vi "rotate_absolute.vi"(3 "error in (no error)":errorcluster, 4 "angle":i32, 5 "revolution":i32) -> (0 "error out":errorcluster)   [LabVIEW 2016]
uses:
  sa commands.ctl
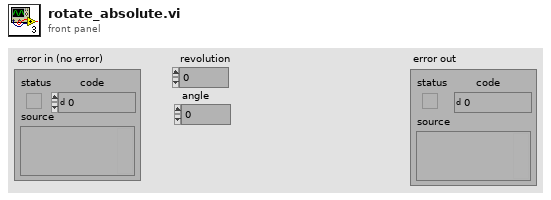
[diagram p1: front panel]
types:
  T1 = typedef "sa commands.ctl" = enum16{"read all", "set system index", "set x channel", "set y channel", "set rotation channel"}
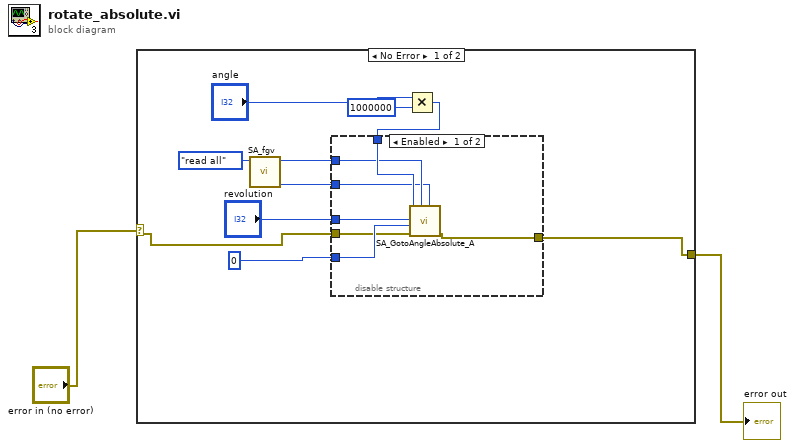
[diagram p0: block diagram]
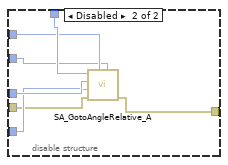
[diagram p2: hidden frame]
diagram:
  n1 = case shown="No Error" "error in (no error)" {
    selector: "error in (no error)" -> [w7 w27]
    tunnel: [w6 w27] -> w1
    frame No Error {
      n2 = call "SA_fgv.vi"("command"=sa_commands."read all") -> ("rotation channel"=w9:u32, "system index"=w10:u32)  [unwired: 3 in, 2 out]
      n3 = Multiply(x="angle", y=1000000) -> (x*y=w4:i32)
      n4 = disable-structure shown="Enabled" {
        disable-tunnel: u32 0 ("holdTime") -> [w19 w22]
        disable-tunnel: "revolution" -> [w18 w23]
        disable-tunnel: w4 -> [w17 w26]
        disable-tunnel: w10 -> [w16 w25]
        disable-tunnel: w9 -> [w15 w24]
        disable-tunnel: w7 -> [w14 w21]
        disable-tunnel: [w13 w20] -> w6
        frame Enabled {
          n5 = call <vilib>:"SA_GotoAngleAbsolute_A.vi"("channelIndex"=w15, "systemIndex"=w16, "error in (no error)"=w14, "holdTime"=w19, "revolution"=w18, "angle"=w17) -> ("error out"=w13:errorcluster)  [unwired: 5 in]
        }
        frame Disabled {
          n6 = call <vilib>:"SA_GotoAngleRelative_A.vi"("channelIndex"=w24, "systemIndex"=w25, "error in (no error)"=w21, "holdTime"=w22, "revolution"=w23, "angleDiff"=w26) -> ("error out"=w20:errorcluster)  [unwired: 5 in]
        }
      }
    }
    frame Error {
    }
  }
  "error out" <- w1
